vi "Accurate Measure With Setting_BU.vi"(0 "DMM ref in":refnum<visa-resource-name>, 1 "channel_count":i32=11, 2 "P_current_count":i32, 3 "N_current_count":i32, 5 "DMM error in":errorcluster, 7 "Accurate Measure Setting":T1, 9 "ESP32 ref in":refnum<visa-resource-name>, 11 "ESP32 error in":errorcluster, 12 "current_mode":u8[](array[numeric])=[0, 0, 0, 0, 0, 0, 0, 0, 0, 0, 0]) -> (4 "DMM ref out":refnum<visa-resource-name>, 6 "DMM error out":errorcluster, 8 "Accurate Data":dbl[](array[numeric]), 10 "ESP32 ref out":refnum<visa-resource-name>, 13 "time_out_count":i32, 14 "Standard Deviation of Data":dbl[](array[numeric]), 15 "ESP32 error out":errorcluster)   [LabVIEW 2023]
uses:
  <instrlib>/Agilent 3446X Series/Agilent 3446X Series.lvlib
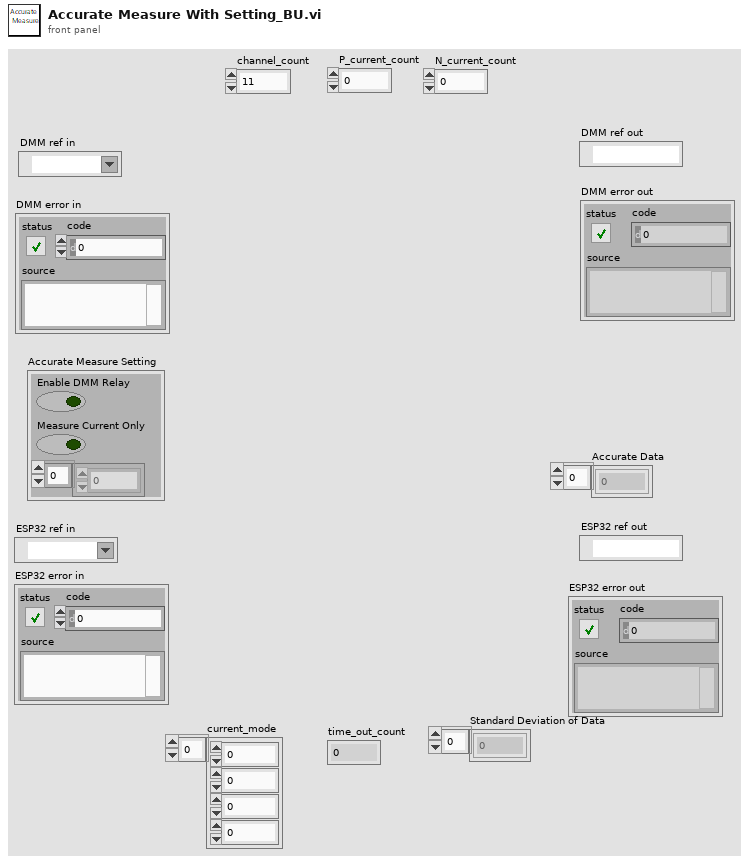
[diagram p1: front panel]
types:
  T1 = cluster{"Enable DMM Relay":bool, "Measure Current Only":bool, dbl[]}
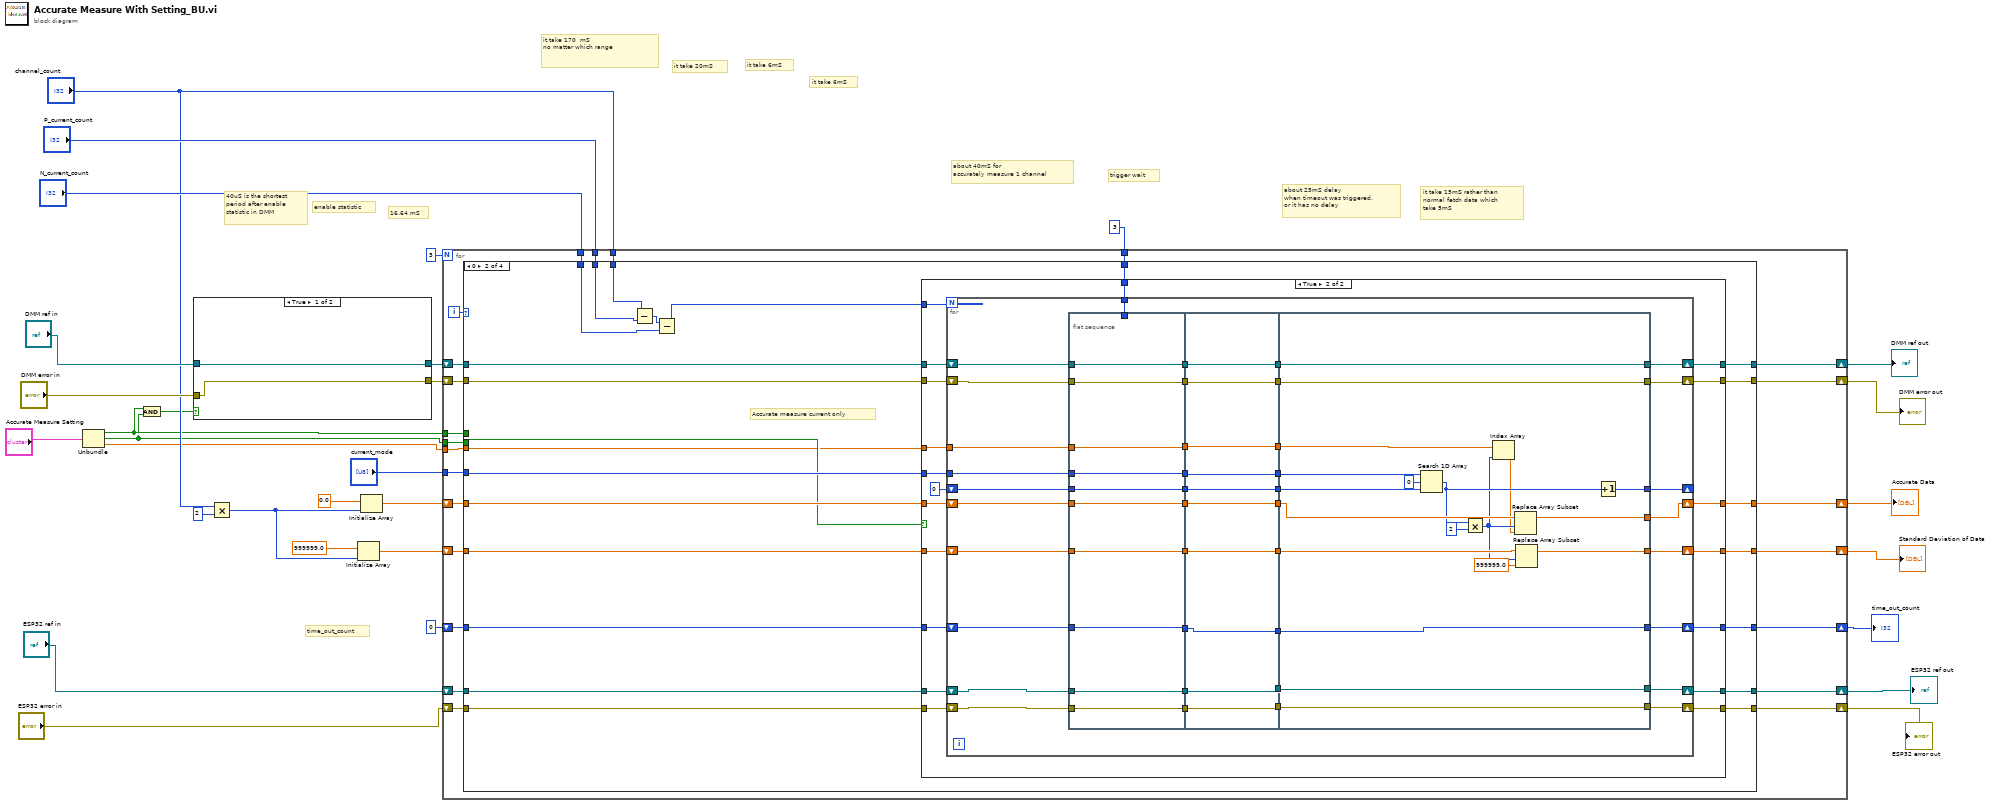
[diagram p0: block diagram]
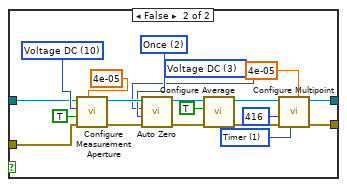
[diagram p2: hidden frame]
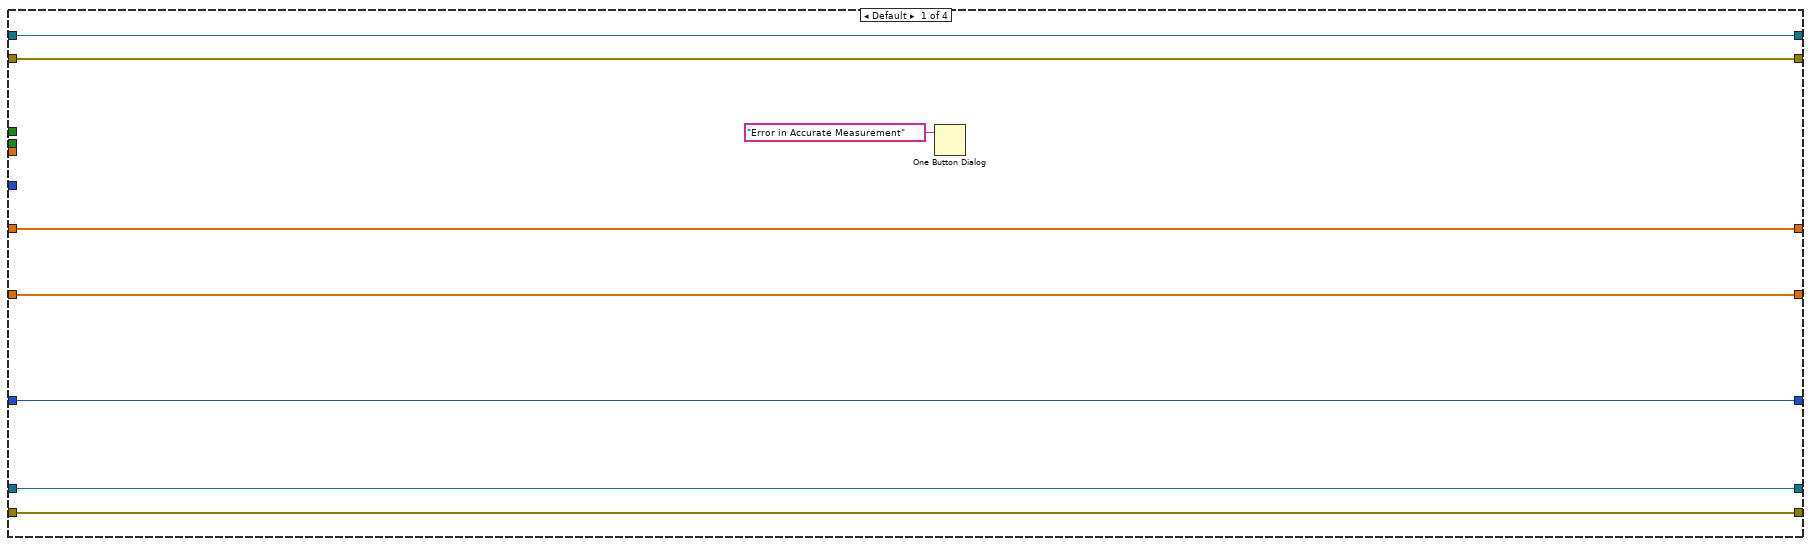
[diagram p3: hidden frame]
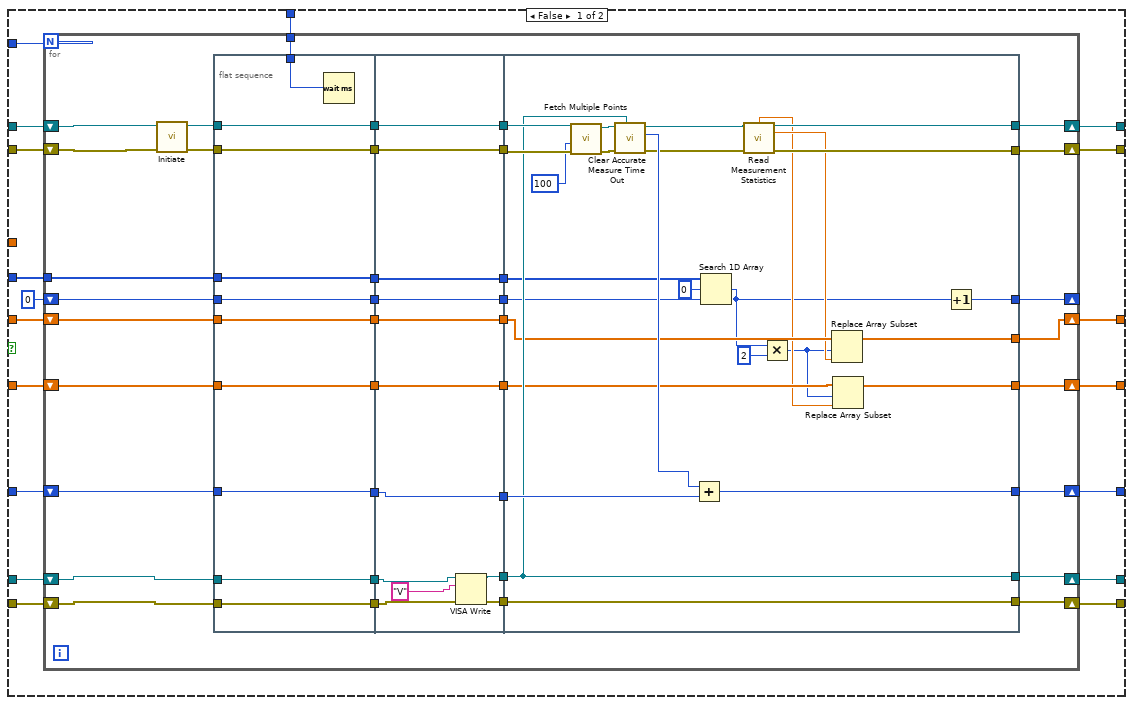
[diagram p4: hidden frame]
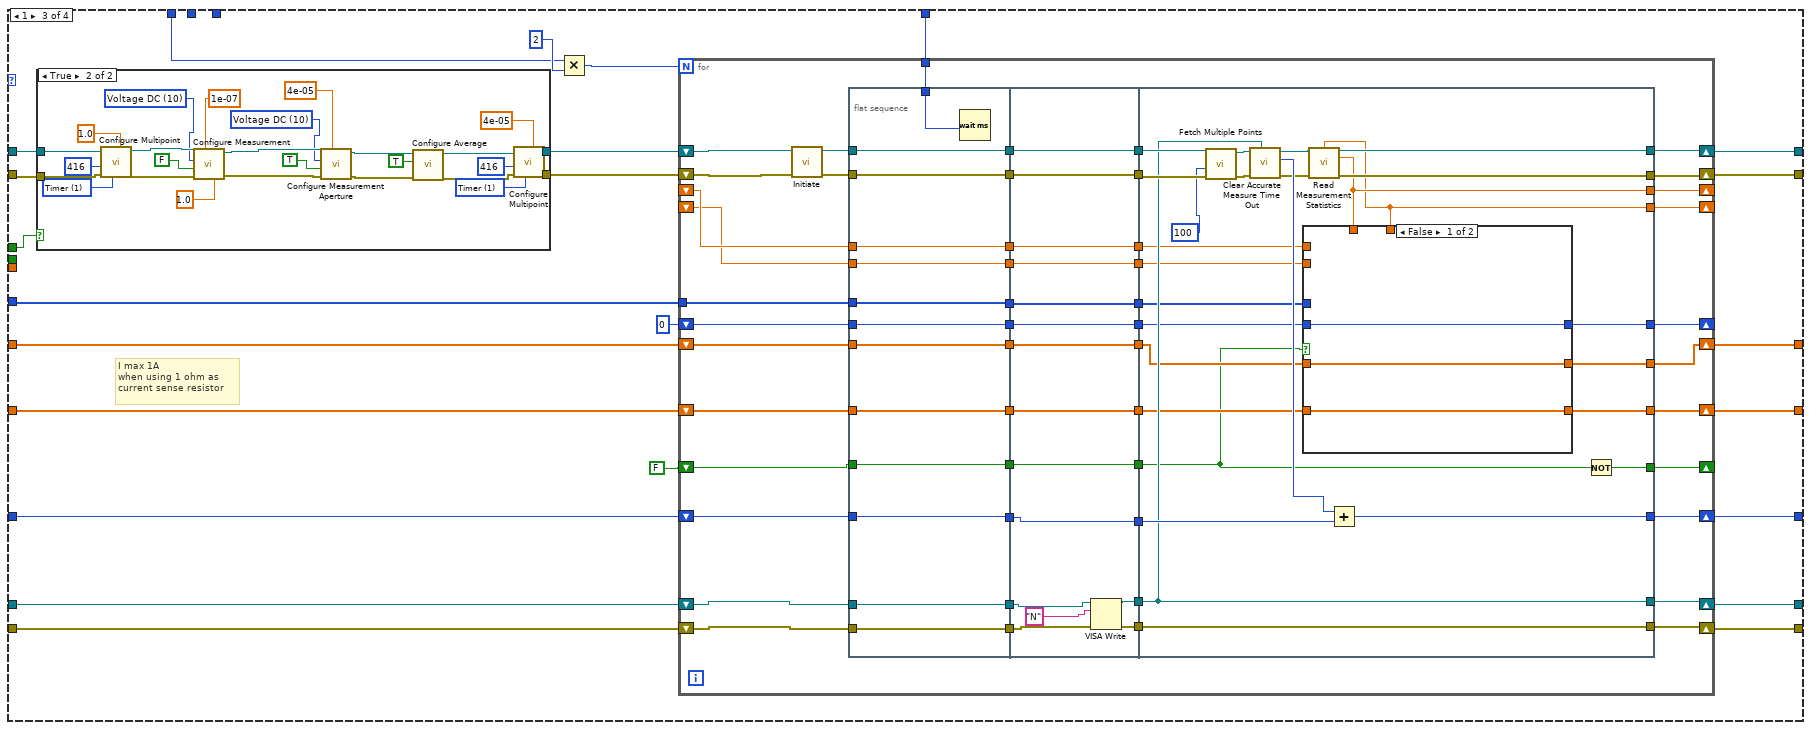
[diagram p5: hidden frame]
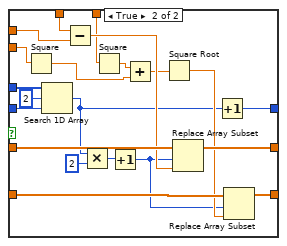
[diagram p7: hidden frame]
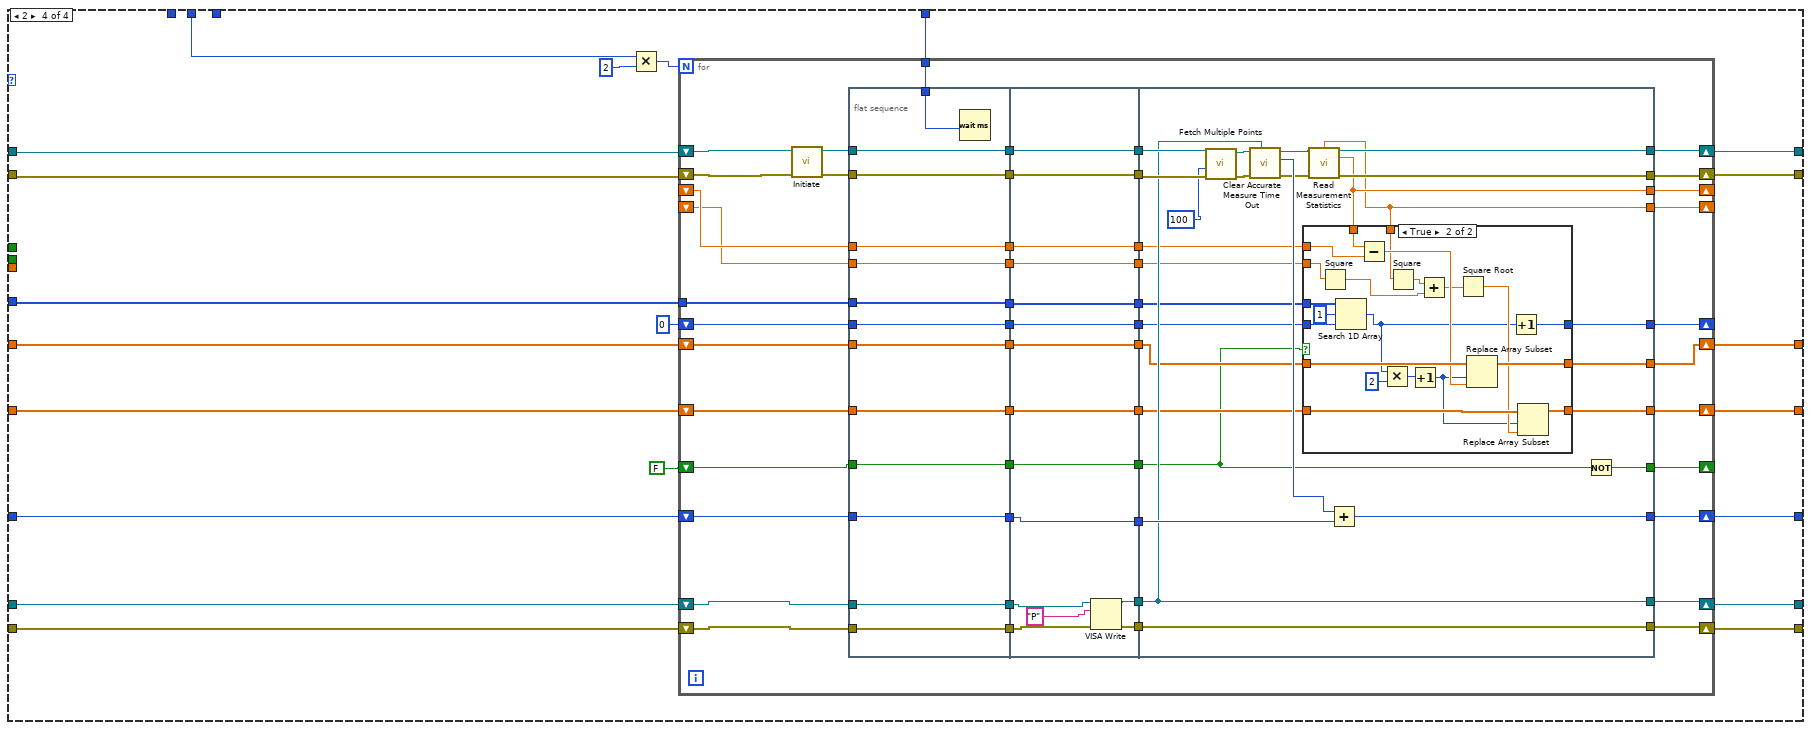
[diagram p8: hidden frame]
diagram:
  # "it take 6mS"
  # "it take 6mS"
  # "it take 20mS"
  # "it take 170  mS\nno matter which range"
  # "it take 15mS rather than\nnormal fetch data which \ntake 5mS"
  # "about 40mS for \naccurately measure 1 channel"
  # "about 25mS delay\nwhen timeout was triggered,\nor it has no delay"
  # "time_out_count"
  # "trigger wait"
  # "16.64 mS"
  # "enable statistic"
  # "40uS is the shortest\nperiod after enable \nstatistic in DMM"
  n1 = Unbundle("Accurate Measure Setting") -> ("Enable DMM Relay"=w3:bool, "Measure Current Only"=w2:bool, w4:dbl[])
  n2 = And(x=w3, y=w2) -> (x .and. y?=w1:bool)
  n3 = case shown="True" w1 {
    tunnel: [w33 w37] -> w31
    tunnel: [w32 w36] -> w30
    tunnel: "DMM ref in" -> [w33 w35]
    tunnel: "DMM error in" -> [w32 w34]
    frame True {
    }
    frame False {
      w39 = 1 items=["Immediate", "Timer"] ("Sample Source (0: Immediate)")
      w46 = 3 items=["Current DC", "Resistance", "Temperature", "Voltage DC"] ("Zero Type (0: Current DC)")
      w47 = 2 items=["Disable", "Enable", "Once"] ("Auto Zero (1: Enable)")
      w43 = 10 items=["Continuity", "Current AC", "Current DC", "Diode", "Frequency", "Resistance 4-wire", "Period", "Resistance 2-wire", "Temperature", "Voltage AC", "Voltage DC", "Voltage DC Ratio", "Capacitance"] ("Measurement Function (0: Continuity)")
      n4 = call <instrlib>:"Configure Measurement Aperture.vi"("Aperture Time (0.1s)"=4e-05, "error in (no error)"=w34, "Enable Aperture (F: Disable)"=TRUE, "Measurement Function (0: Continuity)"=w43, "VISA resource name"=w35) -> ("error out"=w50:errorcluster, "VISA resource name out"=w49:refnum<visa-resource-name>)  [unwired: 5 in]
      n5 = call <instrlib>:"Auto Zero.vi"("error in (no error)"=w50, "Auto Zero (1: Enable)"=w47, "Zero Type (0: Current DC)"=w46, "VISA resource name"=w49) -> ("error out"=w52:errorcluster, "VISA resource name out"=w51:refnum<visa-resource-name>)  [unwired: 6 in]
      n6 = call <instrlib>:"Configure Average.vi"("error in (no error)"=w52, "Enable Statistics (F: Disable)"=TRUE, "VISA resource name"=w51) -> ("error out"=w41:errorcluster, "VISA resource name out"=w42:refnum<visa-resource-name>)  [unwired: 7 in]
      n7 = call <instrlib>:"Configure Multipoint.vi"("Sample Interval (1 Second)"=4e-05, "Sample Source (0: Immediate)"=w39, "error in (no error)"=w41, "Sample Count (1)"=416, "VISA resource name"=w42) -> ("error out"=w36:errorcluster, "VISA resource name out"=w37:refnum<visa-resource-name>)  [unwired: 2 in, 3 out]
    }
  }
  n8 = Multiply(x="channel_count", y=2) -> (x*y=w6:i32)
  n9 = Initialize Array(999999.0 ("Arithmetic Mean"), w6) -> (w16:dbl[])
  n10 = Initialize Array(0.0 ("Arithmetic Mean"), w6) -> (w19:dbl[])
  n11 = for {
    N: 3 -> [_]
    shift-right: [w73] -> w12
    shift-left: "ESP32 ref in" -> [w75]
    shift-right: [w72] -> w11
    shift-left: "ESP32 error in" -> [w74]
    shift-right: [w69] -> w14
    shift-left: w31 -> [w71]
    shift-right: [w68] -> w13
    shift-left: w30 -> [w70]
    tunnel: "channel_count" -> [w67]
    tunnel: "P_current_count" -> [w66]
    tunnel: "N_current_count" -> [w65]
    tunnel: u32 3 ("milliseconds to wait") -> [w64]
    shift-right: [w63] -> w21
    shift-left: 0 -> [w62]
    shift-right: [w56] -> w10
    shift-left: w19 -> [w61]
    tunnel: "current_mode" -> [w60]
    shift-right: [w57] -> w9
    shift-left: w16 -> [w58]
    tunnel: w3 -> [w55]
    tunnel: w2 -> [w54]
    tunnel: w4 -> [w53]
    i -> [w59]
    n12 = case shown="0" w59 {
      tunnel: w75 -> [w81 w102 w332 w510]
      tunnel: w74 -> [w80 w101 w331 w509]
      tunnel: [w81 w98 w328 w506] -> w73
      tunnel: [w80 w97 w327 w505] -> w72
      tunnel: w71 -> [w83 w104 w316 w491]
      tunnel: w70 -> [w82 w103 w315 w490]
      tunnel: [w83 w100 w330 w508] -> w69
      tunnel: [w82 w99 w329 w507] -> w68
      tunnel: w67 -> [_ w96 _ _]
      tunnel: w66 -> [_ w95 _ w493]
      tunnel: w65 -> [_ w94 w311 _]
      tunnel: [w77 w92 w325 w503] -> w63
      tunnel: w64 -> [_ w93 w326 w504]
      tunnel: w62 -> [w77 w91 w324 w502]
      tunnel: w61 -> [w79 w89 w322 w500]
      tunnel: w60 -> [_ w90 w323 w501]
      tunnel: w58 -> [w78 w88 w320 w498]
      tunnel: [w78 w87 w319 w497] -> w57
      tunnel: [w79 w86 w318 w496] -> w56
      tunnel: w55 -> [_ _ w309 _]
      tunnel: w54 -> [_ w85 _ _]
      tunnel: w53 -> [_ w84 _ _]
      frame Default {
        n13 = One Button Dialog(message="Error in Accurate Measurement") -> ()  [unwired: 1 in, 1 out]
      }
      frame 0 {
        # "Accurate measure current only"
        n14 = Subtract(x=w96, y=w95) -> (x-y=w106:i32)
        n15 = Subtract(x=w106, y=w94) -> (x-y=w105:i32)
        n16 = case shown="True" w85 {
          tunnel: w105 -> [w124 w230]
          tunnel: w104 -> [w123 w229]
          tunnel: w103 -> [w122 w228]
          tunnel: w102 -> [w121 w227]
          tunnel: w101 -> [w120 w226]
          tunnel: [w119 w225] -> w100
          tunnel: [w118 w224] -> w99
          tunnel: [w117 w223] -> w98
          tunnel: [w116 w222] -> w97
          tunnel: w93 -> [w115 w221]
          tunnel: [w114 w220] -> w92
          tunnel: w91 -> [w113 w219]
          tunnel: w90 -> [w112 w218]
          tunnel: w89 -> [w111 w217]
          tunnel: w88 -> [w109 w215]
          tunnel: [w108 w214] -> w87
          tunnel: [w107 w213] -> w86
          tunnel: w84 -> [_ w212]
          frame False {
            n17 = for {
              N: w124 -> [_]
              shift-right: [w158] -> w119
              shift-left: w123 -> [w162]
              shift-right: [w157] -> w118
              shift-left: w122 -> [w161]
              shift-right: [w156] -> w117
              shift-left: w121 -> [w160]
              shift-right: [w155] -> w116
              shift-left: w120 -> [w159]
              tunnel: w115 -> [w141]
              shift-right: [w140] -> w114
              shift-left: w113 -> [w154]
              tunnel: w112 -> [w138]
              shift-right: [w126] -> w107
              shift-left: w111 -> [w135]
              shift-right: [w130] -> _
              shift-left: 0 ("index of element") -> [w131]
              shift-right: [w125] -> w108
              shift-left: w109 -> [w128]
              n18 = call <instrlib>:"Initiate.vi"("error in (no error)"=w161, "VISA resource name"=w162) -> ("error out"=w142:errorcluster, "VISA resource name out"=w143:refnum<visa-resource-name>)  [unwired: 8 in]
              n19 = flat-sequence {
                tunnel: [w172] -> w153
                tunnel: w160 -> [w172]
                tunnel: [w171] -> w152
                tunnel: w159 -> [w171]
                tunnel: w143 -> [w170]
                tunnel: [w170] -> w151
                tunnel: [w169] -> w150
                tunnel: w142 -> [w169]
                tunnel: [w168] -> w149
                tunnel: w154 -> [w168]
                tunnel: w141 -> [w167]
                tunnel: [w166] -> w139
                tunnel: w138 -> [w166]
                tunnel: [w165] -> w136
                tunnel: w135 -> [w165]
                tunnel: w131 -> [w164]
                tunnel: [w164] -> w133
                tunnel: [w163] -> w129
                tunnel: w128 -> [w163]
                tunnel: w153 -> [w184]
                tunnel: w152 -> [w183]
                tunnel: w151 -> [w182]
                tunnel: [w182] -> w145
                tunnel: w150 -> [w181]
                tunnel: [w181] -> w146
                tunnel: [w180] -> w147
                tunnel: [w179] -> w148
                tunnel: w149 -> [w177]
                tunnel: [w177] -> w144
                tunnel: w139 -> [w176]
                tunnel: [w176] -> w137
                tunnel: w136 -> [w175]
                tunnel: [w175] -> w134
                tunnel: w133 -> [w174]
                tunnel: [w174] -> w132
                tunnel: w129 -> [w173]
                tunnel: [w173] -> w127
                tunnel: [w211] -> w155
                tunnel: [w199] -> w156
                tunnel: [w203] -> w157
                tunnel: [w204] -> w158
                tunnel: w148 -> [w211]
                tunnel: w147 -> [w199]
                tunnel: w146 -> [w210]
                tunnel: w145 -> [w209]
                tunnel: [w205] -> w140
                tunnel: w144 -> [w200]
                tunnel: w137 -> [w198]
                tunnel: w134 -> [w194]
                tunnel: w132 -> [w196]
                tunnel: [w195] -> w130
                tunnel: w127 -> [w192]
                tunnel: [w190] -> w126
                tunnel: [w189] -> w125
                frame #0 {
                  n20 = Wait (ms)(milliseconds to wait=w167) -> ()  [unwired: 1 out]
                }
                frame #1 {
                  n21 = VISA Write(VISA resource name=w184, write buffer="V" ("data in"), error in (no error)=w183) -> (VISA resource name out=w180:refnum<visa-resource-name>, error out=w179:errorcluster)  [unwired: 1 out]
                }
                frame #2 {
                  n22 = call <instrlib>:"Fetch Multiple Points.vi"("error in (no error)"=w210, "Timeout (10000 ms)"=100, "VISA resource name"=w209) -> ("error out"=w207:errorcluster, "VISA resource name out"=w208:refnum<visa-resource-name>)  [unwired: 1 in, 6 out]
                  n23 = call "Clear Accurate Measure Time Out.vi"("ESP32 ref"=w199, "error in (no error)"=w207, "DMM ref"=w208) -> ("error out"=w201:errorcluster, "Time out count"=w206:i32, "VISA Refnum out"=w202:refnum<visa-resource-name>)  [unwired: 5 in, 1 out]
                  n24 = Add(x=w206, y=w200) -> (x+y=w205:i32)
                  n25 = Search 1D Array(1D array=w198, element=u8 0, start index (0)=w196) -> (index of element=w187:i32)
                  n26 = call <instrlib>:"Read Measurement Statistics.vi"("VISA resource name"=w202, "error in (no error)"=w201) -> ("Standard Deviation"=w191:dbl, "VISA resource name out"=w204:refnum<visa-resource-name>, "Arithmetic Mean"=w193:dbl, "error out"=w203:errorcluster)  [unwired: 6 in, 4 out]
                  n27 = Multiply(x=w187, y=2) -> (x*y=w185:i32)
                  n28 = Replace Array Subset(array=w194, new element=w193, index=w185) -> (w190:dbl[])
                  n29 = Replace Array Subset(array=w192, new element=w191, index=w185) -> (w189:dbl[])
                  n30 = Increment(x=w187) -> (x+1=w195:i32)
                }
              }
            }
          }
          frame True {
            n31 = for {
              N: w230 -> [_]
              shift-right: [w239] -> w225
              shift-left: w229 -> [w241]
              shift-right: [w234] -> w224
              shift-left: w228 -> [w236]
              shift-right: [w267] -> w223
              shift-left: w227 -> [w269]
              shift-right: [w266] -> w222
              shift-left: w226 -> [w268]
              tunnel: w221 -> [w258]
              shift-right: [w257] -> w220
              shift-left: w219 -> [w265]
              tunnel: w218 -> [w255]
              shift-right: [w243] -> w213
              shift-left: w217 -> [w252]
              shift-right: [w247] -> _
              shift-left: 0 ("index of element") -> [w248]
              shift-right: [w242] -> w214
              shift-left: w215 -> [w245]
              tunnel: w212 -> [w231]
              n32 = flat-sequence {
                tunnel: [w279] -> w264
                tunnel: w269 -> [w279]
                tunnel: [w278] -> w263
                tunnel: w268 -> [w278]
                tunnel: [w277] -> w262
                tunnel: w265 -> [w277]
                tunnel: w258 -> [_]
                tunnel: [w276] -> w256
                tunnel: w255 -> [w276]
                tunnel: [w275] -> w253
                tunnel: w252 -> [w275]
                tunnel: w248 -> [w274]
                tunnel: [w274] -> w250
                tunnel: [w273] -> w246
                tunnel: w245 -> [w273]
                tunnel: w241 -> [w272]
                tunnel: [w272] -> w238
                tunnel: [w271] -> w237
                tunnel: w236 -> [w271]
                tunnel: [w270] -> w233
                tunnel: w231 -> [w270]
                tunnel: w264 -> [w282]
                tunnel: w263 -> [w281]
                tunnel: [w282] -> w260
                tunnel: [w281] -> w261
                tunnel: w262 -> [w289]
                tunnel: [w289] -> w259
                tunnel: w256 -> [w288]
                tunnel: [w288] -> w254
                tunnel: w253 -> [w287]
                tunnel: [w287] -> w251
                tunnel: w250 -> [w286]
                tunnel: [w286] -> w249
                tunnel: w246 -> [w285]
                tunnel: [w285] -> w244
                tunnel: [w284] -> w240
                tunnel: w238 -> [w284]
                tunnel: w237 -> [w283]
                tunnel: [w283] -> w235
                tunnel: w233 -> [w280]
                tunnel: [w280] -> w232
                tunnel: [w308] -> w266
                tunnel: [w307] -> w267
                tunnel: w261 -> [w308]
                tunnel: w260 -> [w307]
                tunnel: [w290] -> w257
                tunnel: w259 -> [w290]
                tunnel: w254 -> [w306]
                tunnel: w251 -> [w302]
                tunnel: w249 -> [w304]
                tunnel: [w303] -> w247
                tunnel: w244 -> [w301]
                tunnel: [w300] -> w243
                tunnel: [w299] -> w242
                tunnel: w240 -> [w296]
                tunnel: [w296] -> w239
                tunnel: [w295] -> w234
                tunnel: w235 -> [w295]
                tunnel: w232 -> [w293]
                frame #0 {
                }
                frame #1 {
                }
                frame #2 {
                  n33 = Search 1D Array(1D array=w306, element=u8 0, start index (0)=w304) -> (index of element=w298:i32)
                  n34 = Multiply(x=w298, y=2) -> (x*y=w292:i32)
                  n35 = Index Array(array=w293, index=w292) -> (element=w291:dbl)
                  n36 = Replace Array Subset(array=w302, new element=w291, index=w292) -> (w300:dbl[])
                  n37 = Replace Array Subset(array=w301, new element=999999.0 ("new element/subarray"), index=w292) -> (w299:dbl[])
                  n38 = Increment(x=w298) -> (x+1=w303:i32)
                }
              }
            }
          }
        }
      }
      frame 1 {
        # "I max 1A\nwhen using 1 ohm as \ncurrent sense resistor"
        n39 = case shown="True" w309 {
          tunnel: w316 -> [w334 w340]
          tunnel: w315 -> [w333 w339]
          tunnel: [w334 w338] -> w314
          tunnel: [w333 w337] -> w313
          frame False {
          }
          frame True {
            w350 = 1 items=["Immediate", "Timer"] ("Sample Source (0: Immediate)")
            w346 = 10 items=["Continuity", "Current AC", "Current DC", "Diode", "Frequency", "Resistance 4-wire", "Period", "Resistance 2-wire", "Temperature", "Voltage AC", "Voltage DC", "Voltage DC Ratio", "Capacitance"] ("Measurement Function (0: Continuity)")
            w344 = 1 items=["Immediate", "Timer"] ("Sample Source (0: Immediate)")
            w341 = 10 items=["Continuity", "Current AC", "Current DC", "Diode", "Frequency", "Resistance 4-wire", "Period", "Resistance 2-wire", "Temperature", "Voltage AC", "Voltage DC", "Voltage DC Ratio", "Capacitance"] ("Measurement Function (10: Voltage DC)")
            n40 = call <instrlib>:"Configure Multipoint.vi"("Sample Interval (1 Second)"=1.0, "Sample Source (0: Immediate)"=w344, "error in (no error)"=w339, "Sample Count (1)"=416, "VISA resource name"=w340) -> ("error out"=w357:errorcluster, "VISA resource name out"=w356:refnum<visa-resource-name>)  [unwired: 2 in, 3 out]
            n41 = call <instrlib>:"Configure Measurement.vi"("Manual Range (1)"=1.0, "Absolute Resolution (1E-6)"=1e-07 ("x"), "error in (no error)"=w357, "Auto Range (T: Enable)"=FALSE, "Measurement Function (10: Voltage DC)"=w341, "VISA resource name"=w356) -> ("error out"=w354:errorcluster, "VISA resource name out"=w355:refnum<visa-resource-name>)  [unwired: 4 out]
            n42 = call <instrlib>:"Configure Measurement Aperture.vi"("Aperture Time (0.1s)"=4e-05, "error in (no error)"=w354, "Enable Aperture (F: Disable)"=TRUE, "Measurement Function (0: Continuity)"=w346, "VISA resource name"=w355) -> ("error out"=w359:errorcluster, "VISA resource name out"=w360:refnum<visa-resource-name>)  [unwired: 5 in]
            n43 = call <instrlib>:"Configure Average.vi"("error in (no error)"=w359, "Enable Statistics (F: Disable)"=TRUE, "VISA resource name"=w360) -> ("error out"=w358:errorcluster, "VISA resource name out"=w353:refnum<visa-resource-name>)  [unwired: 7 in]
            n44 = call <instrlib>:"Configure Multipoint.vi"("Sample Interval (1 Second)"=4e-05, "Sample Source (0: Immediate)"=w350, "error in (no error)"=w358, "Sample Count (1)"=416, "VISA resource name"=w353) -> ("error out"=w337:errorcluster, "VISA resource name out"=w338:refnum<visa-resource-name>)  [unwired: 2 in, 3 out]
          }
        }
        n45 = Multiply(x=w311, y=2) -> (x*y=w312:i32)
        n46 = for {
          N: w312 -> [_]
          shift-right: [w406] -> w330
          shift-left: w314 -> [w410]
          shift-right: [w405] -> w329
          shift-left: w313 -> [w409]
          shift-right: [w404] -> w328
          shift-left: w332 -> [w408]
          shift-right: [w403] -> w327
          shift-left: w331 -> [w407]
          tunnel: w326 -> [w389]
          shift-right: [w388] -> w325
          shift-left: w324 -> [w402]
          tunnel: w323 -> [w386]
          shift-right: [w374] -> w318
          shift-left: w322 -> [w383]
          shift-right: [w378] -> _
          shift-left: 0 ("index of element") -> [w379]
          shift-right: [w373] -> w319
          shift-left: w320 -> [w376]
          shift-right: [w369] -> _
          shift-left: FALSE ("Enable Statistics (F: Disable)") -> [w370]
          shift-right: [w368] -> _
          shift-left: _ -> [w366]
          shift-right: [w367] -> _
          shift-left: _ -> [w363]
          n47 = call <instrlib>:"Initiate.vi"("error in (no error)"=w409, "VISA resource name"=w410) -> ("error out"=w390:errorcluster, "VISA resource name out"=w391:refnum<visa-resource-name>)  [unwired: 8 in]
          n48 = flat-sequence {
            tunnel: [w423] -> w401
            tunnel: w408 -> [w423]
            tunnel: [w422] -> w400
            tunnel: w407 -> [w422]
            tunnel: w391 -> [w421]
            tunnel: [w421] -> w399
            tunnel: [w420] -> w398
            tunnel: w390 -> [w420]
            tunnel: [w419] -> w397
            tunnel: w402 -> [w419]
            tunnel: w389 -> [w418]
            tunnel: [w417] -> w387
            tunnel: w386 -> [w417]
            tunnel: [w416] -> w384
            tunnel: w383 -> [w416]
            tunnel: w379 -> [w415]
            tunnel: [w415] -> w381
            tunnel: [w414] -> w377
            tunnel: w376 -> [w414]
            tunnel: w370 -> [w413]
            tunnel: [w413] -> w372
            tunnel: w366 -> [w412]
            tunnel: [w412] -> w364
            tunnel: w363 -> [w411]
            tunnel: [w411] -> w362
            tunnel: w401 -> [w438]
            tunnel: w400 -> [w437]
            tunnel: w399 -> [w436]
            tunnel: [w436] -> w393
            tunnel: w398 -> [w435]
            tunnel: [w435] -> w394
            tunnel: [w434] -> w395
            tunnel: [w433] -> w396
            tunnel: w397 -> [w431]
            tunnel: [w431] -> w392
            tunnel: w387 -> [w430]
            tunnel: [w430] -> w385
            tunnel: w384 -> [w429]
            tunnel: [w429] -> w382
            tunnel: w381 -> [w428]
            tunnel: [w428] -> w380
            tunnel: w377 -> [w427]
            tunnel: [w427] -> w375
            tunnel: w372 -> [w426]
            tunnel: [w426] -> w371
            tunnel: [w425] -> w365
            tunnel: w364 -> [w425]
            tunnel: w362 -> [w424]
            tunnel: [w424] -> w361
            tunnel: [w465] -> w403
            tunnel: [w453] -> w404
            tunnel: [w457] -> w405
            tunnel: [w458] -> w406
            tunnel: w396 -> [w465]
            tunnel: w395 -> [w453]
            tunnel: w394 -> [w464]
            tunnel: w393 -> [w463]
            tunnel: [w459] -> w388
            tunnel: w392 -> [w454]
            tunnel: w385 -> [w452]
            tunnel: w382 -> [w449]
            tunnel: w380 -> [w451]
            tunnel: [w450] -> w378
            tunnel: w375 -> [w448]
            tunnel: [w447] -> w374
            tunnel: [w446] -> w373
            tunnel: w371 -> [w445]
            tunnel: [w444] -> w369
            tunnel: [w441] -> w368
            tunnel: [w440] -> w367
            tunnel: w365 -> [w443]
            tunnel: w361 -> [w442]
            frame #0 {
              n49 = Wait (ms)(milliseconds to wait=w418) -> ()  [unwired: 1 out]
            }
            frame #1 {
              n50 = VISA Write(VISA resource name=w438, write buffer="N" ("data in"), error in (no error)=w437) -> (VISA resource name out=w434:refnum<visa-resource-name>, error out=w433:errorcluster)  [unwired: 1 out]
            }
            frame #2 {
              n51 = call <instrlib>:"Fetch Multiple Points.vi"("error in (no error)"=w464, "Timeout (10000 ms)"=100, "VISA resource name"=w463) -> ("error out"=w461:errorcluster, "VISA resource name out"=w462:refnum<visa-resource-name>)  [unwired: 1 in, 6 out]
              n52 = call "Clear Accurate Measure Time Out.vi"("ESP32 ref"=w453, "error in (no error)"=w461, "DMM ref"=w462) -> ("error out"=w455:errorcluster, "Time out count"=w460:i32, "VISA Refnum out"=w456:refnum<visa-resource-name>)  [unwired: 5 in, 1 out]
              n53 = call <instrlib>:"Read Measurement Statistics.vi"("VISA resource name"=w456, "error in (no error)"=w455) -> ("Standard Deviation"=w440:dbl, "VISA resource name out"=w458:refnum<visa-resource-name>, "Arithmetic Mean"=w441:dbl, "error out"=w457:errorcluster)  [unwired: 6 in, 4 out]
              n54 = case shown="False" w445 {
                tunnel: w452 -> [_ w489]
                tunnel: w451 -> [w468 w487]
                tunnel: [w468 w486] -> w450
                tunnel: w449 -> [w467 w485]
                tunnel: w448 -> [w466 w484]
                tunnel: [w467 w483] -> w447
                tunnel: [w466 w482] -> w446
                tunnel: w443 -> [_ w473]
                tunnel: w442 -> [_ w480]
                tunnel: w441 -> [_ w474]
                tunnel: w440 -> [_ w479]
                frame False {
                }
                frame True {
                  n55 = Square(x=w480) -> (x^2=w477:dbl)
                  n56 = Search 1D Array(1D array=w489, element=u8 2, start index (0)=w487) -> (index of element=w470:i32)
                  n57 = Subtract(x=w474, y=w473) -> (x-y=w481:dbl)
                  n58 = Multiply(x=w470, y=2) -> (x*y=w471:i32)
                  n59 = Square(x=w479) -> (x^2=w478:dbl)
                  n60 = Increment(x=w471) -> (x+1=w469:i32)
                  n61 = Add(x=w478, y=w477) -> (x+y=w476:dbl)
                  n62 = Square Root(x=w476) -> (sqrt(x)=w475:dbl)
                  n63 = Replace Array Subset(array=w485, new element=w481, index=w469) -> (w483:dbl[])
                  n64 = Increment(x=w470) -> (x+1=w486:i32)
                  n65 = Replace Array Subset(array=w484, new element=w475, index=w469) -> (w482:dbl[])
                }
              }
              n66 = Add(x=w460, y=w454) -> (x+y=w459:i32)
              n67 = Not(x=w445) -> (.not. x?=w444:bool)
            }
          }
        }
      }
      frame 2 {
        n68 = Multiply(x=w493, y=2) -> (x*y=w492:i32)
        n69 = for {
          N: w492 -> [_]
          shift-right: [w556] -> w508
          shift-left: w491 -> [w560]
          shift-right: [w555] -> w507
          shift-left: w490 -> [w559]
          shift-right: [w554] -> w506
          shift-left: w510 -> [w558]
          shift-right: [w553] -> w505
          shift-left: w509 -> [w557]
          tunnel: w504 -> [w539]
          shift-right: [w538] -> w503
          shift-left: w502 -> [w552]
          tunnel: w501 -> [w536]
          shift-right: [w524] -> w496
          shift-left: w500 -> [w533]
          shift-right: [w528] -> _
          shift-left: 0 ("index of element") -> [w529]
          shift-right: [w523] -> w497
          shift-left: w498 -> [w526]
          shift-right: [w519] -> _
          shift-left: FALSE ("Enable Statistics (F: Disable)") -> [w520]
          shift-right: [w518] -> _
          shift-left: _ -> [w516]
          shift-right: [w517] -> _
          shift-left: _ -> [w513]
          n70 = call <instrlib>:"Initiate.vi"("error in (no error)"=w559, "VISA resource name"=w560) -> ("error out"=w540:errorcluster, "VISA resource name out"=w541:refnum<visa-resource-name>)  [unwired: 8 in]
          n71 = flat-sequence {
            tunnel: [w573] -> w551
            tunnel: w558 -> [w573]
            tunnel: [w572] -> w550
            tunnel: w557 -> [w572]
            tunnel: w541 -> [w571]
            tunnel: [w571] -> w549
            tunnel: [w570] -> w548
            tunnel: w540 -> [w570]
            tunnel: [w569] -> w547
            tunnel: w552 -> [w569]
            tunnel: w539 -> [w568]
            tunnel: [w567] -> w537
            tunnel: w536 -> [w567]
            tunnel: [w566] -> w534
            tunnel: w533 -> [w566]
            tunnel: w529 -> [w565]
            tunnel: [w565] -> w531
            tunnel: [w564] -> w527
            tunnel: w526 -> [w564]
            tunnel: w520 -> [w563]
            tunnel: [w563] -> w522
            tunnel: w516 -> [w562]
            tunnel: [w562] -> w514
            tunnel: w513 -> [w561]
            tunnel: [w561] -> w512
            tunnel: w551 -> [w588]
            tunnel: w550 -> [w587]
            tunnel: w549 -> [w586]
            tunnel: [w586] -> w543
            tunnel: w548 -> [w585]
            tunnel: [w585] -> w544
            tunnel: [w584] -> w545
            tunnel: [w583] -> w546
            tunnel: w547 -> [w581]
            tunnel: [w581] -> w542
            tunnel: w537 -> [w580]
            tunnel: [w580] -> w535
            tunnel: w534 -> [w579]
            tunnel: [w579] -> w532
            tunnel: w531 -> [w578]
            tunnel: [w578] -> w530
            tunnel: w527 -> [w577]
            tunnel: [w577] -> w525
            tunnel: w522 -> [w576]
            tunnel: [w576] -> w521
            tunnel: [w575] -> w515
            tunnel: w514 -> [w575]
            tunnel: w512 -> [w574]
            tunnel: [w574] -> w511
            tunnel: [w615] -> w553
            tunnel: [w603] -> w554
            tunnel: [w607] -> w555
            tunnel: [w608] -> w556
            tunnel: w546 -> [w615]
            tunnel: w545 -> [w603]
            tunnel: w544 -> [w614]
            tunnel: w543 -> [w613]
            tunnel: [w609] -> w538
            tunnel: w542 -> [w604]
            tunnel: w535 -> [w602]
            tunnel: w532 -> [w599]
            tunnel: w530 -> [w601]
            tunnel: [w600] -> w528
            tunnel: w525 -> [w598]
            tunnel: [w597] -> w524
            tunnel: [w596] -> w523
            tunnel: w521 -> [w595]
            tunnel: [w594] -> w519
            tunnel: [w591] -> w518
            tunnel: [w590] -> w517
            tunnel: w515 -> [w593]
            tunnel: w511 -> [w592]
            frame #0 {
              n72 = Wait (ms)(milliseconds to wait=w568) -> ()  [unwired: 1 out]
            }
            frame #1 {
              n73 = VISA Write(VISA resource name=w588, write buffer="P" ("data in"), error in (no error)=w587) -> (VISA resource name out=w584:refnum<visa-resource-name>, error out=w583:errorcluster)  [unwired: 1 out]
            }
            frame #2 {
              n74 = call <instrlib>:"Fetch Multiple Points.vi"("error in (no error)"=w614, "Timeout (10000 ms)"=100, "VISA resource name"=w613) -> ("error out"=w611:errorcluster, "VISA resource name out"=w612:refnum<visa-resource-name>)  [unwired: 1 in, 6 out]
              n75 = call "Clear Accurate Measure Time Out.vi"("ESP32 ref"=w603, "error in (no error)"=w611, "DMM ref"=w612) -> ("error out"=w605:errorcluster, "Time out count"=w610:i32, "VISA Refnum out"=w606:refnum<visa-resource-name>)  [unwired: 5 in, 1 out]
              n76 = call <instrlib>:"Read Measurement Statistics.vi"("VISA resource name"=w606, "error in (no error)"=w605) -> ("Standard Deviation"=w590:dbl, "VISA resource name out"=w608:refnum<visa-resource-name>, "Arithmetic Mean"=w591:dbl, "error out"=w607:errorcluster)  [unwired: 6 in, 4 out]
              n77 = case shown="True" w595 {
                tunnel: w602 -> [_ w639]
                tunnel: w601 -> [w618 w637]
                tunnel: [w618 w636] -> w600
                tunnel: w599 -> [w617 w635]
                tunnel: w598 -> [w616 w634]
                tunnel: [w617 w633] -> w597
                tunnel: [w616 w632] -> w596
                tunnel: w593 -> [_ w623]
                tunnel: w592 -> [_ w630]
                tunnel: w591 -> [_ w624]
                tunnel: w590 -> [_ w629]
                frame False {
                }
                frame True {
                  n78 = Square(x=w630) -> (x^2=w627:dbl)
                  n79 = Search 1D Array(1D array=w639, element=u8 1, start index (0)=w637) -> (index of element=w620:i32)
                  n80 = Subtract(x=w624, y=w623) -> (x-y=w631:dbl)
                  n81 = Multiply(x=w620, y=2) -> (x*y=w621:i32)
                  n82 = Square(x=w629) -> (x^2=w628:dbl)
                  n83 = Increment(x=w621) -> (x+1=w619:i32)
                  n84 = Add(x=w628, y=w627) -> (x+y=w626:dbl)
                  n85 = Square Root(x=w626) -> (sqrt(x)=w625:dbl)
                  n86 = Replace Array Subset(array=w635, new element=w631, index=w619) -> (w633:dbl[])
                  n87 = Increment(x=w620) -> (x+1=w636:i32)
                  n88 = Replace Array Subset(array=w634, new element=w625, index=w619) -> (w632:dbl[])
                }
              }
              n89 = Add(x=w610, y=w604) -> (x+y=w609:i32)
              n90 = Not(x=w595) -> (.not. x?=w594:bool)
            }
          }
        }
      }
    }
  }
  "time_out_count" <- w21
  "DMM ref out" <- w14
  "DMM error out" <- w13
  "ESP32 ref out" <- w12
  "ESP32 error out" <- w11
  "Accurate Data" <- w10
  "Standard Deviation of Data" <- w9
